vi "Copy_Proj_Data.vi"(8 "error in (no error)":errorcluster, 9 "IB_Destination.lvclass":refnum<class "IB_Destination.lvclass">, 10 "IB_Tree_Item_Proj in":refnum<class "IB_Tree_Item_Proj.lvclass">, 11 "IB_EXE in":refnum<class "IB_EXE.lvclass">) -> (0 "error out":errorcluster, 3 "IB_EXE out":refnum<class "IB_EXE.lvclass">)   [LabVIEW 2020, in "IB_EXE.lvclass"]
uses:
  <vilib>/AppBuilder/IB_Classes/Source/Container/Build/EXE/IB_EXE.lvclass
  <vilib>/AppBuilder/IB_Classes/Source/Container/Build/EXE/IB_EXE.lvclass/IB_EXE.ctl
  <vilib>/AppBuilder/IB_Classes/Source/Container/Build/IB_Source_Build.lvclass
  <vilib>/AppBuilder/IB_Classes/Source/Container/IB_Source_Container.lvclass
  <vilib>/AppBuilder/IB_Classes/Source/IB_Source.lvclass
  <vilib>/AppBuilder/IB_Classes/Source/File/CtrFile/IB_CtrFile.lvclass
  <vilib>/AppBuilder/IB_Classes/Shortcut/IB_Shortcut.lvclass
  <vilib>/AppBuilder/IB_Classes/Installer/Installer.lvclass
  e:/builds/penguin/labview/branches/2020/dev/dist/vi.lib/AppBuilder/IB_Classes/Source/Container/Build/IB_Source_Build.lvclass
  e:/builds/penguin/labview/branches/2020/dev/dist/vi.lib/AppBuilder/IB_Classes/Source/Container/IB_Source_Container.lvclass
  e:/builds/penguin/labview/branches/2020/dev/dist/vi.lib/AppBuilder/IB_Classes/Source/IB_Source.lvclass
  e:/builds/penguin/labview/branches/2020/dev/dist/vi.lib/AppBuilder/IB_Classes/Source/Container/Build/EXE/IB_EXE.lvclass
  e:/builds/penguin/labview/branches/2020/dev/dist/vi.lib/AppBuilder/IB_Classes/Source/File/IB_Source_File.lvclass
  e:/builds/penguin/labview/branches/2020/dev/dist/vi.lib/AppBuilder/IB_Classes/Source/File/CtrFile/IB_CtrFile.lvclass
  <vilib>/AppBuilder/IB_Classes/Tree_Item_Proj/IB_Tree_Item_Proj.lvclass
  <vilib>/AppBuilder/IB_Classes/Destination/IB_Destination.lvclass
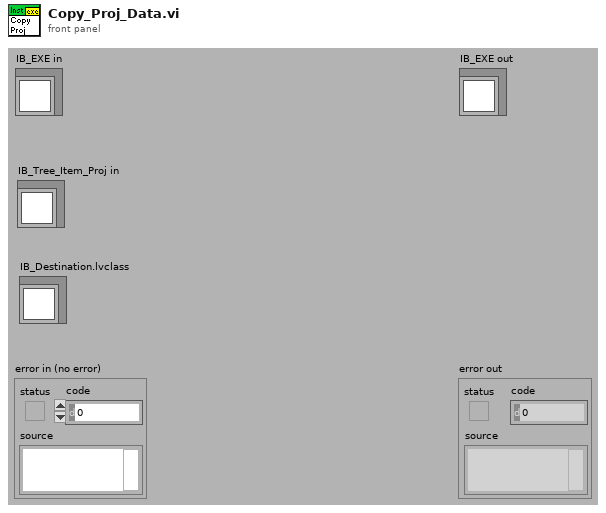
[diagram p1: front panel]
types:
  T1 = typedef "IB_Source_Container.ctl" = cluster{"files":refnum<class "IB_CtrFile.lvclass">[], "previewed?":bool, "preview error?":bool}
  T2 = typedef "IB_Source.ctl" = cluster{"name":string, "sourceTag":string, "destTag":string, "path":path, "eng_installPath":string, "UI_inBuild?":bool, "str ref?":bool}
  T3 = typedef "IB_Installer.ctl" = cluster{"Destination":refnum<class "IB_Destination.lvclass">[], "Source":refnum<class "IB_Source.lvclass">[], "buildObject":T4, "defaultDir":string, "platform":string, "author":string, "productName":string, "buildSpecName":string, "hide":bool, "requireLVDevSys":bool, "autoIncrement":bool, "includeError":bool, "readmeID":string, "buildLocation":path, "readmePath":path, "mediaSize":u16, "language":T5, "productVersion":T6, "preview":bool, "programmatic":bool, "progressBarEvents":T7, "userLog_Path":path, "shortcutAddresses":T9[], "EXE_Install Address":string, "EXE_Uninstall Address":string, "additional NIPaths":refnum<class "Dest_NI_NIPath.lvclass">[], "web service itemIDs":string[], "installerName":string}
  T4 = typedef "ItemRef.ctl" = u64
  T5 = typedef "CDK_sTypeDef_Languages.ctl" = u16
  T6 = typedef "CDK_sTypeDef_ProductVersion.ctl" = cluster{"Major":u8, "Minor":u8, "Update":u16}
  T7 = typedef "provcom_ProgressBar_Events.ctl" = cluster{"newJob":refnum<user-event>, "newItem":refnum<user-event>, "errorMsg":T8, "cancel":refnum<user-event>}
  T8 = typedef "mxLvBuildError.ctl" = refnum<user-event>
  T9 = typedef "CDK_sTypeDef_ShortcutAddress.ctl" = cluster{"file":string, "shortcut":string}
  T10 = typedef "IB_Shortcut.ctl" = cluster{"name":string, "destIndex":i32, "subDir":string, "address":string}
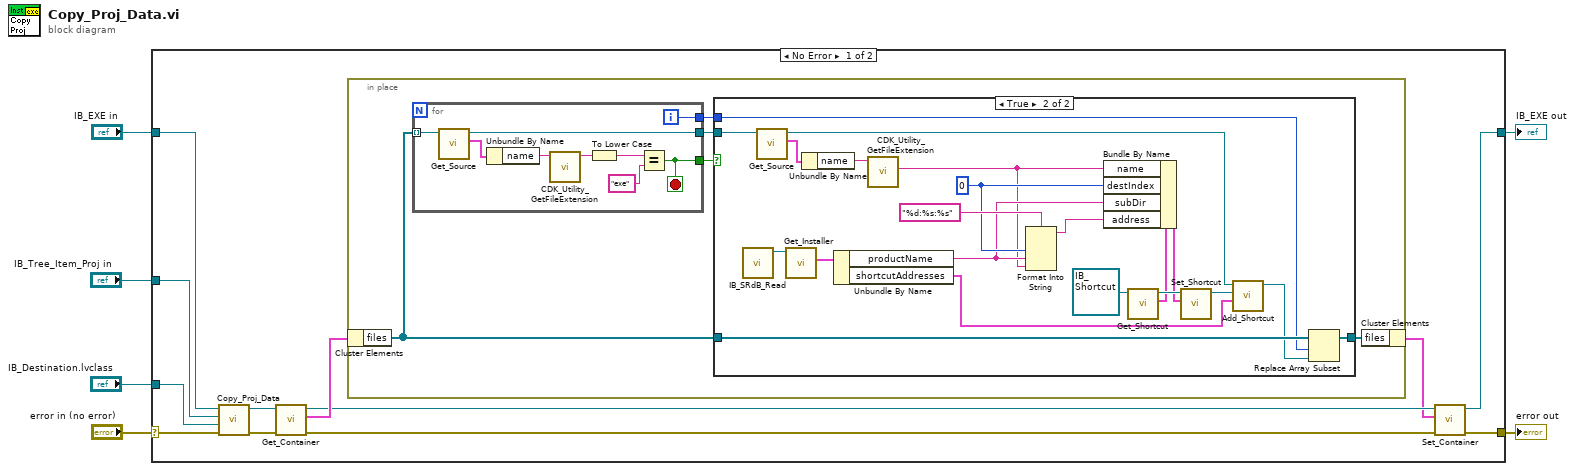
[diagram p0: block diagram]
diagram:
  n1 = case shown="No Error" "error in (no error)" {
    selector: "error in (no error)" -> [w13 w56]
    tunnel: "IB_Destination.lvclass" -> [w18 _]
    tunnel: "IB_Tree_Item_Proj in" -> [w17 _]
    tunnel: "IB_EXE in" -> [w16 w55]
    tunnel: [w10 w55] -> w3
    tunnel: [w8 w56] -> w2
    frame No Error {
      n2 = call-parent "Copy_Proj_Data.vi"("error in (no error)"=w13, "IB_Destination.lvclass"=w18, "IB_Tree_Item_Proj in"=w17, "IB_Source_Build in"=w16) -> ("error out"=w14:errorcluster, "IB_Source_Build out"=w15:refnum<class "IB_EXE.lvclass">)  [unwired: 6 out]
      n3 = call <vilib>:"Get_Container.vi"("error in (no error)"=w14, "IB_Source_Container in"=w15) -> ("error out"=w9:errorcluster, "data"=w12:T1, "IB_Source_Container out"=w11:refnum<class "IB_EXE.lvclass">)  [unwired: 7 out]
      n4 = in-place {
        n5 = in-place-cluster #1(w12) -> ("files"=w23:refnum<class "IB_CtrFile.lvclass">[])
        n6 = for {
          tunnel: w23 -> [w54] mode=indexing
          tunnel: [w48] -> w21
          tunnel: [w47] -> w20
          tunnel: [w46] -> w19
          i -> [w48]
          stop <- w47 stop-if-true
          n7 = call <vilib>:"Get_Source.vi"("IB_Source in"=w54) -> ("data"=w53:T2, "IB_Source out"=w46:refnum<class "IB_CtrFile.lvclass">)  [unwired: 1 in, 8 out]
          n8 = Unbundle By Name(w53) -> ("name"=w51:string)
          n9 = call <resource>:"CDK_Utility_GetFileExtension.vi"("filename"=w51) -> ("extension"=w52:string)  [unwired: 10 out]
          n10 = To Lower Case(string=w52) -> (all lower case string=w50:string)
          n11 = Equal?(x=w50, y="exe") -> (x = y?=w47:bool)
        }
        n12 = case shown="True" w20 {
          tunnel: w23 -> [w24 w45]
          tunnel: [w24 w44] -> w22
          tunnel: w21 -> [_ w43]
          tunnel: w19 -> [_ w32]
          frame False {
          }
          frame True {
            w28 = u16 0 ("Value")
            n13 = call <resource>:"IB_SRdB_Read.vi"() -> ("installer out"=w41:refnum<class "Installer.lvclass">)  [unwired: 1 in, 10 out]
            n14 = call <vilib>:"Get_Source.vi"("IB_Source in"=w32) -> ("data"=w39:T2, "IB_Source out"=w31:refnum<class "IB_CtrFile.lvclass">)  [unwired: 1 in, 8 out]
            n15 = call <vilib>:"Get_Installer.vi"("Installer in"=w41) -> ("data"=w38:T3)  [unwired: 1 in, 9 out]
            n16 = Unbundle By Name(w39) -> ("name"=w40:string)
            n17 = Unbundle By Name(w38) -> ("productName"=w27:string, "shortcutAddresses"=w30:T9[])
            n18 = call <resource>:"CDK_Utility_GetFileExtension.vi"("filename"=w40) -> ("filename w/o extension"=w26:string)  [unwired: 10 out]
            n19 = Format Into String(format string="%d:%s:%s", w28, w27, w26) -> (resulting string=w25:string)  [unwired: 2 in, 1 out]
            n20 = call <vilib>:"Get_Shortcut.vi"("Class in"=refnum<class "IB_Shortcut.lvclass"> refnum ("IB_Shortcut.lvclass")) -> ("data"=w34:T10, "Class out"=w36:refnum<class "IB_Shortcut.lvclass">)  [unwired: 1 in, 8 out]
            n21 = Bundle By Name(cluster=w34, "name"=w26, "destIndex"=w28, "subDir"=w27, "address"=w25) -> (w35:T10)
            n22 = call <vilib>:"Set_Shortcut.vi"("data"=w35, "Class in"=w36) -> ("Class out"=w33:refnum<class "IB_Shortcut.lvclass">)  [unwired: 1 in, 8 out]
            n23 = call-dynamic "Add_Shortcut.vi"("shortcutAddresses"=w30, "shortcut"=w33, "IB_Source_File in"=w31) -> ("IB_Source_File out"=w42:refnum<class "IB_CtrFile.lvclass">)  [unwired: 1 in, 7 out]
            n24 = Replace Array Subset(array=w45, new element=w42, index=w43) -> (w44:refnum<class "IB_CtrFile.lvclass">[])
          }
        }
        n25 = in-place-cluster #1("files"=w22) -> (w7:T1)
      }
      n26 = call <vilib>:"Set_Container.vi"("error in (no error)"=w9, "data"=w7, "IB_Source_Container in"=w11) -> ("error out"=w8:errorcluster, "IB_Source_Container out"=w10:refnum<class "IB_EXE.lvclass">)  [unwired: 7 out]
    }
    frame Error {
    }
  }
  "error out" <- w2
  "IB_EXE out" <- w3
